vi "timeoutMicrosecondsToMclks.vi"(1 "vcsel_period_pclks":u8, 2 "timeout_period_us":u32) -> (0 "timeout_period_mclks":u32)   [LabVIEW 2018]
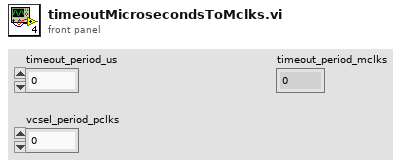
[diagram p1: front panel]
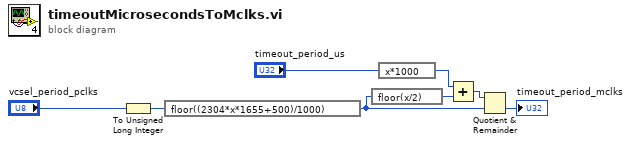
[diagram p0: block diagram]
diagram:
  n1 = To Unsigned Long Integer(number="vcsel_period_pclks") -> (unsigned 32bit integer=w8:u32)
  n2 = expression code="floor((2304*x*1655+500)/1000)"(w8) -> (w2:u32)
  n3 = expression code="floor(x/2)"(w2) -> (w5:u32)
  n4 = expression code="x*1000"("timeout_period_us") -> (w4:u32)
  n5 = Add(x=w4, y=w5) -> (x+y=w3:u32)
  n6 = Quotient & Remainder(x=w3, y=w2) -> (floor(x/y)=→"timeout_period_mclks":u32)  [unwired: 1 out]
